vi "ReformatFitFormula.vi"(0 "Current Fit Formula":string, 1 "Curve Fit Index":i32, 2 "Variables":string[](array[string]), 3 "Channel Names":string[](array[string]), 4 "X Axis Full Ch Name":string) -> (5 "Reformatted Current Fit Formula":string)   [LabVIEW 2015]
doc: "Given the Current Fit Formula, the curve fit of interest (specified by the Curve Fit Index), the Variables String Array, and the corresponding Channel Names Array, Reformat the Current Fit Formula String to be amenable to Results File Plotter Metadata Channel \"Maths\" text format. Specifically, variables are replaced with <<Full:Channel:Names>> and \"**\" is replaced with \"^\" to signify exponentiation."
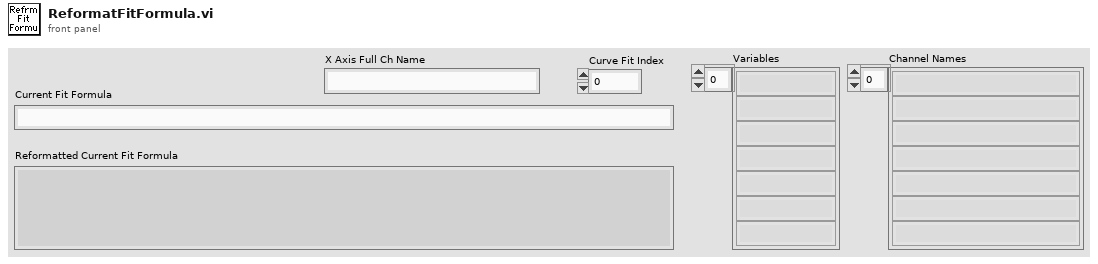
[diagram p1: front panel]
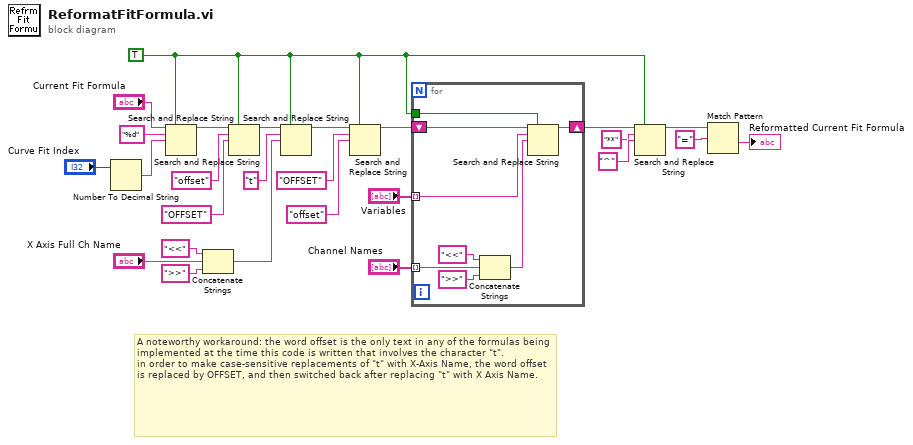
[diagram p0: block diagram]
diagram:
  w1 = TRUE ("replace all? (F)")
  # "A noteworthy workaround: the word offset is the only text in any of the formulas being implemented at the time this code is written that involves the character \"t\".\nin order to make case-sensitive replacements of \"t\" with X-Axis Name, the word offset is replaced by OFFSET, and then switched back after replacing \"t\" with X Axis Name."
  n1 = Number To Decimal String(number="Curve Fit Index") -> (decimal integer string=w22:string)  [unwired: 1 in]
  n2 = Search and Replace String(replace all?=w1, input string="Current Fit Formula", search string="%d", replace string=w22) -> (result string=w16:string)  [unwired: 4 in, 3 out]
  n3 = Concatenate Strings("<<" ("string"), "X Axis Full Ch Name", ">>" ("string")) -> (w12:string)
  n4 = Search and Replace String(replace all?=w1, input string=w16, search string="offset", replace string="OFFSET" ("replace string (\"\")")) -> (result string=w7:string)  [unwired: 4 in, 3 out]
  n5 = Search and Replace String(replace all?=w1, input string=w7, search string="t", replace string=w12) -> (result string=w13:string)  [unwired: 4 in, 3 out]
  n6 = Search and Replace String(replace all?=w1, input string=w13, search string="OFFSET", replace string="offset" ("replace string (\"\")")) -> (result string=w6:string)  [unwired: 4 in, 3 out]
  n7 = for {
    tunnel: "Variables" -> [w31] mode=indexing
    tunnel: "Channel Names" -> [w30] mode=indexing
    shift-right: [w27] -> w3
    shift-left: w6 -> [w29]
    tunnel: w1 -> [w28]
    n8 = Concatenate Strings("<<" ("string"), w30, ">>" ("string")) -> (w32:string)
    n9 = Search and Replace String(replace all?=w28, input string=w29, search string=w31, replace string=w32) -> (result string=w27:string)  [unwired: 4 in, 3 out]
  }
  n10 = Search and Replace String(replace all?=w1, input string=w3, search string="**", replace string="^" ("replace string (\"\")")) -> (result string=w2:string)  [unwired: 4 in, 3 out]
  n11 = Match Pattern(string=w2, regular expression="=") -> (after substring=→"Reformatted Current Fit Formula":string)  [unwired: 1 in, 3 out]
